vi "DUT_Dialog.vi"() -> (1 "DUT out":i32, 2 "Cancelled":bool)   [LabVIEW 2022 SP3, in "DUT_Handler_Simple.lvlib" / "DUT_Handler_Simple.lvclass"]
uses:
  DUT_Handler_Simple.lvclass
panel:
  in  "DUT":i32=1 caption="String" min=1 max=6
  in  "OK":bool caption="Blank"
  in  "Cancel":bool caption="Blank"
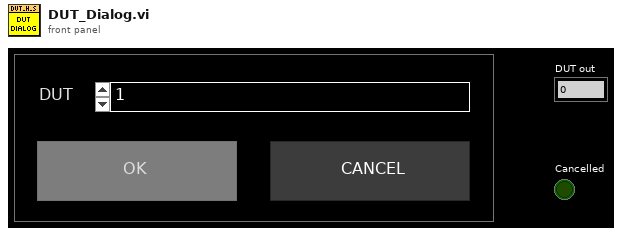
[diagram p1: front panel]
types:
  T1 = enum8{"Enabled", "Disabled", "Disabled and Grayed Out"}
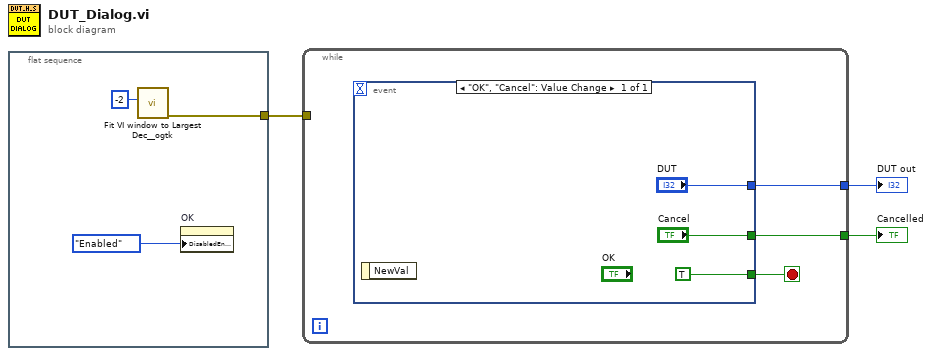
[diagram p0: block diagram]
diagram:
  n1 = flat-sequence {
    tunnel: [w4] -> w1
    frame #0 {
      n2 = call <userlib>:"Fit VI window to Largest Dec__ogtk.vi"("border spacing (2 px)"=-2) -> ("error out"=w4:errorcluster)  [unwired: 5 in, 1 out]
      n3 = property on="OK" class="Bool"("DisabledEnum"=T1."Enabled" ("Disabled")) -> ()  [unwired: 2 in, 2 out]
    }
  }
  n4 = while {
    tunnel: [w8] -> w3
    tunnel: [w7] -> w2
    tunnel: w1 -> [_]
    stop <- w9 stop-if-true
    n5 = event shown="[0] \"OK\", \"Cancel\": Value Change" {
      selector: _ -> [_]
      dyn-events: _ -> [_]
      timeout: _ -> [_]
      tunnel: [TRUE ("OK")] -> w9
      tunnel: ["Cancel"] -> w8
      tunnel: ["DUT"] -> w7
      event "OK", "Cancel": Value Change {
        n6 = event-data() -> ()  [unwired: 1 in, 1 out]
      }
    }
  }
  "Cancelled" <- w3
  "DUT out" <- w2
